vi "RESTful Load Template.vi"(8 "error in (no error)":errorcluster) -> (0 "error out":errorcluster, 3 "INI File Template":string)   [LabVIEW 2020]
doc: "This VI contains or load the default output template."
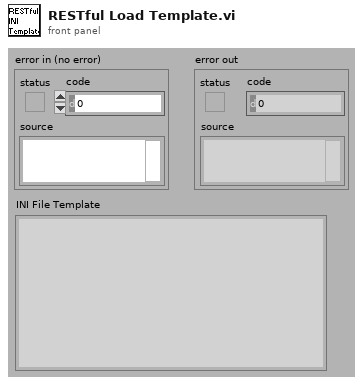
[diagram p1: front panel]
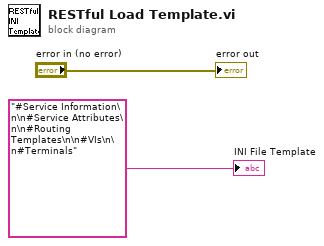
[diagram p0: block diagram]
diagram:
  "INI File Template" <- "#Service Information\n\n#Service Attributes\n\n#Routing Templates\n\n#VIs\n\n#Terminals" ("INI File Template")
  "error out" <- "error in (no error)"
